vi "dvp Vi Set Color Solution Sel.vi"(10 "ColorSolutionSel":u32, 11 "handle":u32) -> (3 "function return":u32(ring))   [LabVIEW 2018, in "LabViewDVPCamera.lvlib"]
doc: "LabviewDvp2Api dvpStatus dvpViSetColorSolutionSel(dvpHandle handle, dvpUint32 ColorSolutionSel);"
uses:
  LabViewDVPCamera.lvlib
  LabViewDVPCamera/LabViewDVPCamera.dll
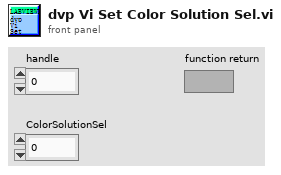
[diagram p1: front panel]
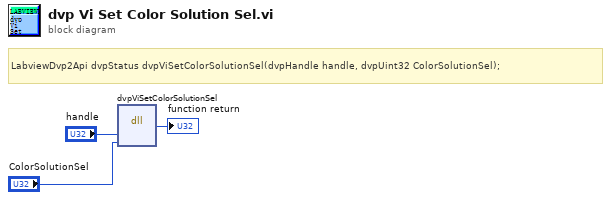
[diagram p0: block diagram]
diagram:
  # "LabviewDvp2Api dvpStatus dvpViSetColorSolutionSel(dvpHandle handle, dvpUint32 ColorSolutionSel);"
  n1 = dll-call lib="C:/Program Files (x86)/DVP2 Labview cn 64/Sample/LabViewDVPCamera/LabViewDVPCamera.*" fn="dvpViSetColorSolutionSel"("handle"="handle", "ColorSolutionSel"="ColorSolutionSel") -> (→"function return":u32)  [unwired: 5 in, 2 out]
